vi "Set Quantity.vi"(6 "Backend engine":T1, 8 "error in":errorcluster, 11 "Quantity":T2={"Name"="A", "Value"=[[1.0]], "Uncertainty"=[[1.0]], "Degrees of\nFreedom"=[[10.0]], "Correlation"=[[10.0]], "Randomized uncertainty"=[[10.0]]}) -> (0 "error out":errorcluster)   [LabVIEW 2013]
doc: "Set Quantity."
uses:
  TD Quantity.ctl
  TD Backend Engine.ctl
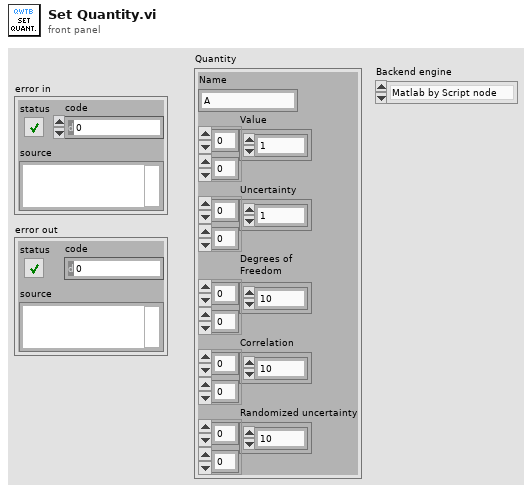
[diagram p1: front panel]
types:
  T1 = typedef "TD Backend Engine.ctl" = enum16{"Matlab by Script node", "GNU Octave by GOLPI"}
  T2 = typedef "TD Quantity.ctl" = cluster{"Name":string, "Value":dbl[][], "Uncertainty":dbl[][], "Degrees of\nFreedom":dbl[][], "Correlation":dbl[][], "Randomized uncertainty":dbl[][]}
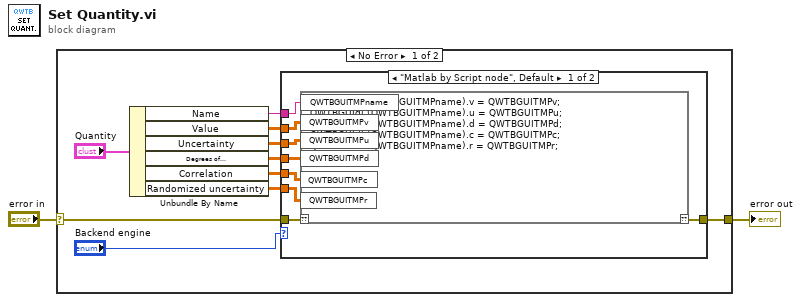
[diagram p0: block diagram]
diagram:
  n1 = case shown="No Error" "error in" {
    selector: "error in" -> [w10 w22]
    tunnel: [w11 w22] -> w2
    frame No Error {
      n2 = Unbundle By Name("Quantity") -> ("Name"=w8:string, "Value"=w7:dbl[][], "Uncertainty"=w12:dbl[][], "Degrees of\nFreedom"=w6:dbl[][], "Correlation"=w5:dbl[][], "Randomized uncertainty"=w4:dbl[][])
      n3 = case shown="\"Matlab by Script node\", Default" "Backend engine" {
        tunnel: w12 -> [w20 _]
        tunnel: [w19 w21] -> w11
        tunnel: w10 -> [w18 w21]
        tunnel: w8 -> [w17 _]
        tunnel: w7 -> [w16 _]
        tunnel: w6 -> [w15 _]
        tunnel: w5 -> [w14 _]
        tunnel: w4 -> [w13 _]
        frame "Matlab by Script node", Default {
          n4 = script code="QWTBGUIdi.(QWTBGUITMPname).v = QWTBGUITMPv;\nQWTBGUIdi.(QWTBGUITMPname).u = QWTBGUITMPu;\nQWTBGUIdi.(QWTBGUITMPname).d = QWTBGUITMPd;\nQWTBGUIdi.(QWTBGUITMPname).c = QWTBGUITMPc;\nQWTBGUIdi.(QWTBGUITMPname).r = QWTBGUITMPr;"("??"=w18, "QWTBGUITMPv"=w16, "QWTBGUITMPu"=w20, "QWTBGUITMPd"=w15, "QWTBGUITMPname"=w17, "QWTBGUITMPc"=w14, "QWTBGUITMPr"=w13) -> ("??"=w19:errorcluster)
        }
        frame "GNU Octave by GOLPI" {
          # "#2do"
        }
      }
    }
    frame Error {
    }
  }
  "error out" <- w2
